vi "LM model function multi magnetometer.vi"(3 "output control":T1, 4 "data":variant, 5 "X":dbl[](array[numeric]), 6 "a":dbl[](array[numeric])) -> (0 "error out":errorcluster, 1 "f'(X,a)":dbl[][](array[numeric]), 2 "f(X,a)":dbl[](array[numeric]))   [LabVIEW 2017]
doc: "This template is the starting point for creating a model function to be passed to the Nonlinear Curve Fit.vi."
uses:
  <vilib>/gmath/NumericalOptimization/LM_output select.ctl
  typedefs/magnetomter reading set.ctl
  <vilib>/gmath/NI_Gmath.lvlib
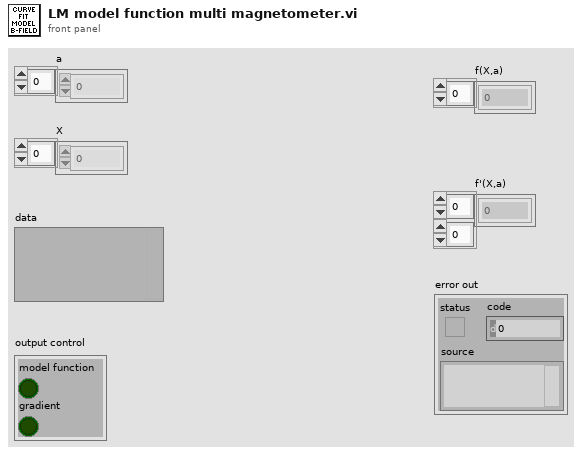
[diagram p1: front panel]
types:
  T1 = typedef "NI_Gmath.lvlib/LM_output select.ctl" = cluster{"model function":bool, "gradient":bool}
  T2 = typedef "magnetomter reading set.ctl" = cluster{"time":fxp<+,48,48>, "mag readings":cluster{"magnetometer index":dbl, "Bx":dbl, "By":dbl, "Bz":dbl, "magnetometer x":dbl, "magnetometer y":dbl}[]}
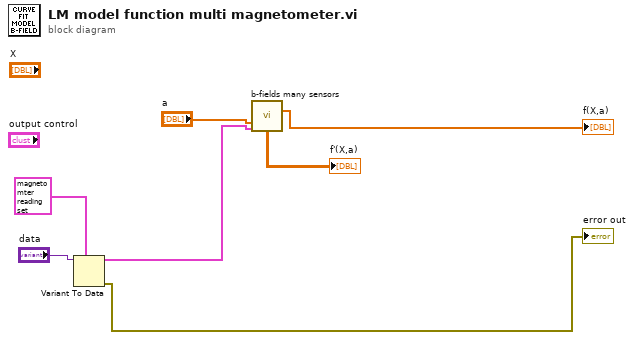
[diagram p0: block diagram]
diagram:
  n1 = Variant To Data(type=T2 {"time"=0.0, "mag readings"=[]} ("Magnetometer reading set"), Variant="data") -> (data=w3:T2, error out=→"error out":errorcluster)  [unwired: 1 in]
  n2 = call "b-fields many sensors.vi"("param vector in"="a", "Magnetometer reading set"=w3) -> ("pf - flat"=→"f(X,a)":dbl[], "derivative"=→"f'(X,a)":dbl[][])  [unwired: 7 in, 5 out]
